vi "Define Test.vi"(8 "error in":errorcluster, 11 "Label (VI Title)":string) -> (0 "error out":errorcluster, 2 "Properties.Test":refnum<class "Properties.Test.lvclass">)   [LabVIEW 2021, in "Banana.Caraya.lvlib" / "Platano.CarayaTestSuite.lvclass"]
uses:
  Platano.CarayaTestSuite.lvclass
  <vilib>/addons/_JKI Toolkits/Caraya/classes/Properties.Test/Properties.Test.lvclass
  C:/Program Files (x86)/National Instruments/LabVIEW 2021/vi.lib/addons/_JKI Toolkits/Caraya/classes/Properties/Properties.lvclass
  Bananas/Banana/Banana.lvclass/Banana.ctl
  <vilib>/LabVIEW Open Source Project/Data Manipulation/Variant/Variant_SetName.vi
  <vilib>/LabVIEW Open Source Project/Data Manipulation/Variant/Variant_BuildClusterFromElementArray.vi
  Bananas/Banana/Read Ephemerals.vi
  <vilib>/LabVIEW Open Source Project/Data Manipulation/Variant/Variant_EmptyCluster.vi
  Bananas/DefineTest/DefineTest.lvclass
  C:/Repositories/LVOS/Bananas/lv-src/Bananas/BananaPeel/BananaPeel.lvclass
  <vilib>/LabVIEW Open Source Project/Data Manipulation/Variant/Variant_ListElements.vi
  <vilib>/LabVIEW Open Source Project/Data Manipulation/TypeDescriptor/TypeDescriptor_SetName.vi
  <vilib>/Utility/GetType.llb/TD_Create Cluster.vi
  Bananas/DefineSuite/DefineSuite.lvclass
  Bananas/DestroySuite/DestroySuite.lvclass
  Bananas/BananaPeel/BananaPeel.lvclass
  Platano.CarayaTestSuite.lvclass/Platano.CarayaTestSuite.ctl
  <vilib>/addons/_JKI Toolkits/Caraya/classes/Test/Test.lvclass
  Bananas/Platano/Platano.lvclass
  Bananas/Banana/Banana.lvclass
  Bananas/Leaf/Leaf.lvclass
  Leaf.Properties.Test/Leaf.Properties.Test.lvclass
  C:/Repositories/LVOS/Bananas/lv-src/Banana.Caraya/Leaf.Properties/Leaf.Properties.lvclass
  C:/Repositories/LVOS/Bananas/lv-src/Bananas/Leaf/Leaf.lvclass
  C:/Repositories/LVOS/Bananas/lv-src/Bananas/Leaf.TestCase/Leaf.TestCase.lvclass
  C:/Repositories/LVOS/Bananas/lv-src/Banana.Caraya/Leaf.Properties.Test/Leaf.Properties.Test.lvclass
  C:/Repositories/LVOS/Bananas/lv-src/Bananas/DefineTest/DefineTest.lvclass
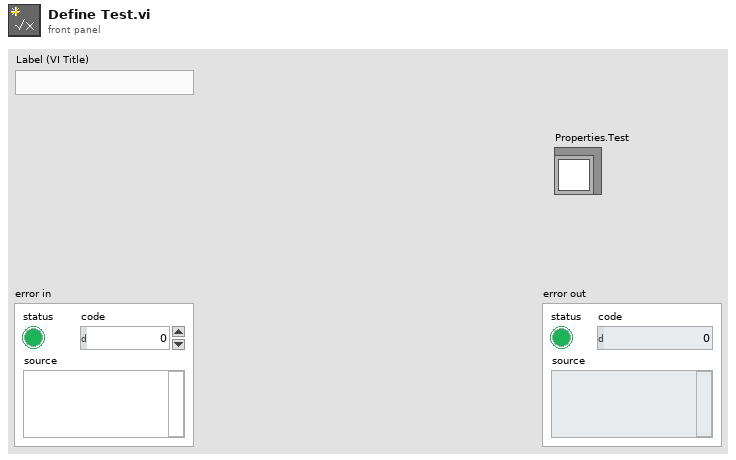
[diagram p1: front panel]
types:
  T1 = typedef "Bananas.lvlib/Test Strategies -- cluster.ctl" = cluster{"DefineTest":refnum<class "DefineTest.lvclass">, "DefineSuite":refnum<class "DefineSuite.lvclass">, "DestroySuite":refnum<class "DestroySuite.lvclass">}
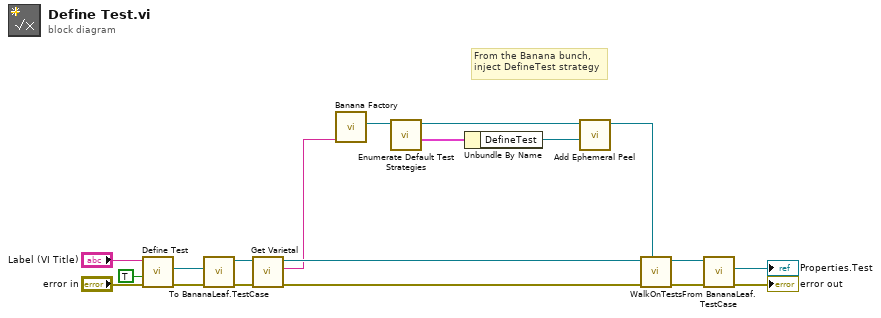
[diagram p0: block diagram]
diagram:
  # "From the Banana bunch,\ninject DefineTest strategy"
  n1 = call <vilib>:"Define Test.vi"("error in (no error)"="error in", "Register with caller (F)"=TRUE, "Label (VI Title)"="Label (VI Title)") -> ("error out"=w7:errorcluster, "Properties.Test"=w4:refnum<class "Properties.Test.lvclass">)  [unwired: 7 in]
  n2 = call "To BananaLeaf.TestCase.vi"("Properties.Test"=w4) -> ("Leaf.Properties.TestCase out"=w3:refnum<class "Leaf.Properties.Test.lvclass">)  [unwired: 10 in]
  n3 = call "Get Varietal.vi"("error in (no error)"=w7, "Leaf in"=w3) -> ("error out"=w6:errorcluster, "Varietal"=w5:string, "Leaf out"=w8:refnum<class "Leaf.Properties.Test.lvclass">)  [unwired: 7 in]
  n4 = call "Banana Factory.vi"("Varietal"=w5) -> ("Banana"=w9:refnum<class "Banana.lvclass">)  [unwired: 9 in, 1 out]
  n5 = call "Enumerate Default Test Strategies.vi"("Banana"=w9) -> ("Strategies"=w11:T1, "Banana"=w10:refnum<class "Banana.lvclass">)  [unwired: 9 in]
  n6 = Unbundle By Name(w11) -> ("DefineTest"=w13:refnum<class "DefineTest.lvclass">)
  n7 = call "Add Ephemeral Peel.vi"("BananaPeel"=w13, "Banana"=w10) -> ("Banana"=w12:refnum<class "Banana.lvclass">)  [unwired: 9 in]
  n8 = call "WalkOnTests.vi"("Banana"=w12, "error in (no error)"=w6, "Leaf.TestCase"=w8) -> ("error out"=→"error out":errorcluster, "Leaf.TestCase"=w2:refnum<class "Leaf.Properties.Test.lvclass">)  [unwired: 7 in]
  n9 = call "From BananaLeaf.TestCase.vi"("Leaf.Properties.TestCase"=w2) -> ("Properties.Test"=→"Properties.Test":refnum<class "Properties.Test.lvclass">)  [unwired: 10 in]
